vi "raise Height set.vi"(8 "error in (no error)":errorcluster, 10 "Height_cm":dbl) -> (0 "error out":errorcluster)   [LabVIEW 2019]
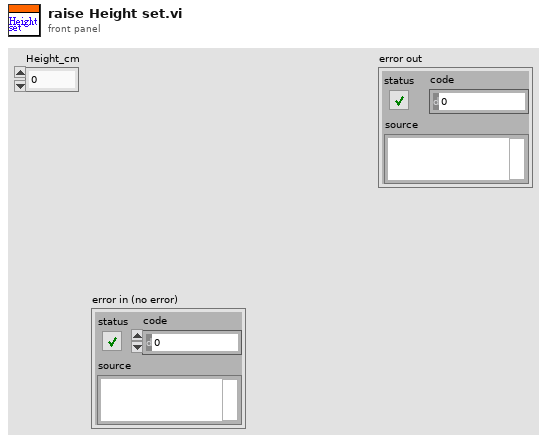
[diagram p1: front panel]
types:
  T1 = cluster{"read mode":enum16{"polling", "blocking"}, "write mode":enum16{"polling", "blocking"}}
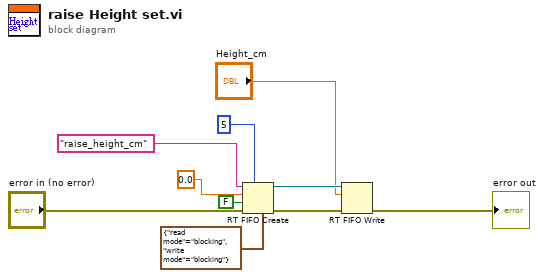
[diagram p0: block diagram]
diagram:
  n1 = RT FIFO Create(0:"raise_height_cm" ("name (unnamed)"), 1:0.0, 2:FALSE ("create if not found? (T)"), 3:"error in (no error)", 4:u32 5 ("size (10)"), 7:T1 {"read mode"=enum."blocking", "write mode"=enum."blocking"} ("r/w modes (polling,polling)")) -> (8:w8:refnum<k33>, 11:w9:errorcluster)  [unwired: 2 in, 1 out]
  n2 = RT FIFO Write(0:w8, 1:"Height_cm", 3:w9) -> (11:→"error out":errorcluster)  [unwired: 2 in, 3 out]
